vi "Alpha Ver 2.0.vi"() -> ()   [LabVIEW 2015]
uses:
  <instrlib>/Keithley 622x LV 2009/Utility/Typedefs/KE622x -- Instrument Type.ctl
  <instrlib>/Keithley 622x LV 2009/Keithley 622x.lvlib
panel:
  out "concatenated string":string
  out "write buffer":string="*RST\nSOUR:PDEL:HIGH 1e-3\nSOUR:PDEL:LOW 0\nSOUR:PDEL:WIDT 500e-6\nSOUR:PDEL:SDEL 100e-6\nSOUR:PDEL:COUN INF\nSOUR:PDEL:RANG BEST\nSOUR:PDEL:INT 5\nSOUR:PDEL:LME 2\nTRAC:POIN 200\nSOUR:PDEL:ARM\nINIT:IMM"
  out "LM_com":string
  out "I_com":string
  out "R_com":string
  out "C_com":string
  out "SD_com":string
  out "W_com":string
  out "LL_com":string
  out "HL_com":string
  in  "INF Button":bool
  in  "prefix 2":u16(ring)
  in  "prefix":u16(ring)
  in  "Low Measure":u16(ring)=1 items=["1", "2"]
  in  "Interval":dbl=5.0 min=5.0 max=999999.0 step=1.0
  in  "Ranging":string(combo)="BEST"
  in  "Count":dbl=1.0 min=1.0 max=65536.0 step=1.0
  in  "Source Delay":dbl
  in  "Width":dbl
  in  "Low Level":dbl min=-0.105 max=0.105
  in  "High Level":dbl
  out "2182A \nconnected ?":string
  in  "STOP":bool
  out "Measurement\nUnits":string
  out "2182A Voltage \nRange":string
  out "error out":errorcluster
  # "Pulse Measurement System"
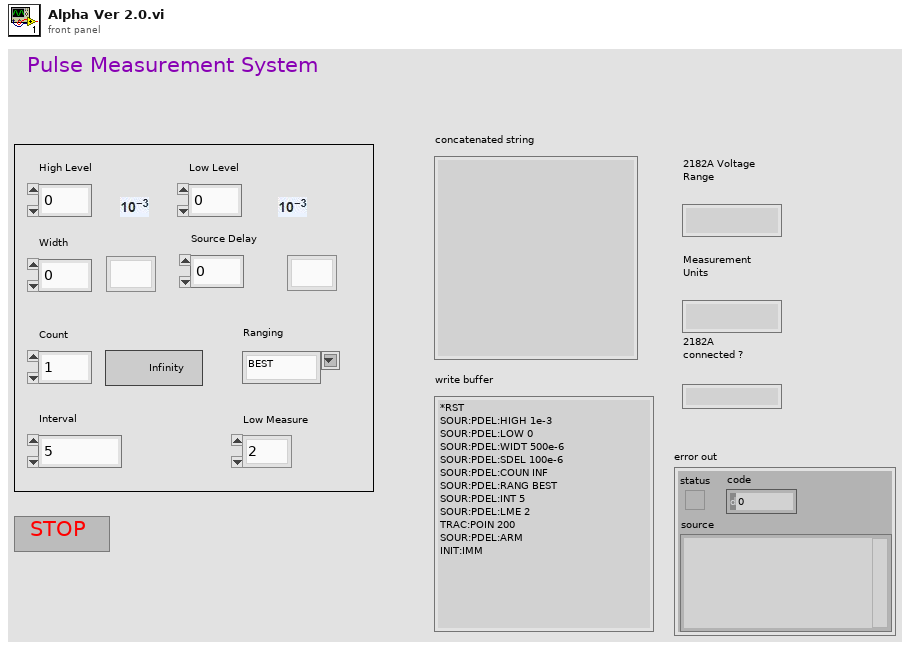
[diagram p1: front panel]
types:
  T1 = typedef "Keithley 622x.lvlib/KE622x -- Instrument Type.ctl" = enum16{"KE6220", "KE6221"}
  T2 = cluster{"VISA resource name out":refnum<visa-resource-name>, "error out":errorcluster}
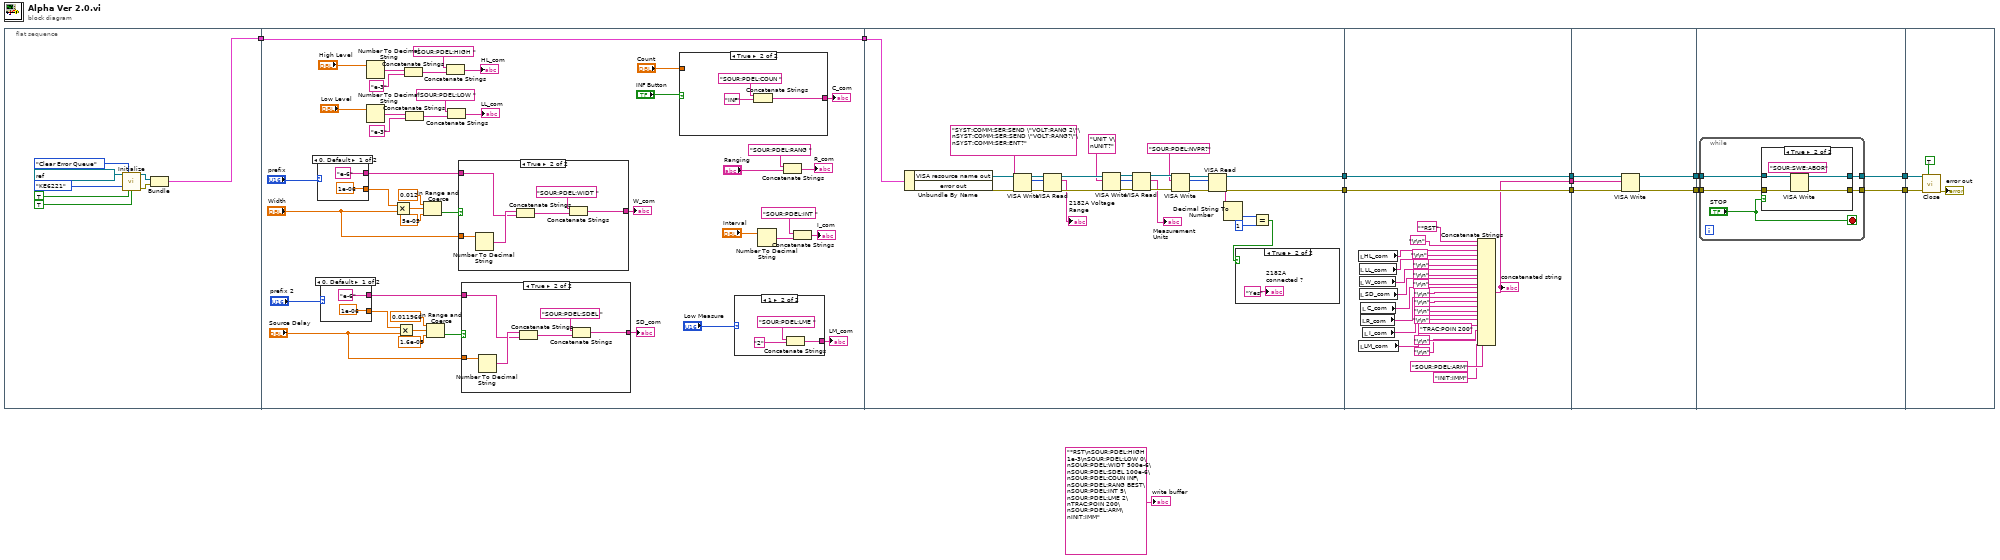
[diagram p0: block diagram]
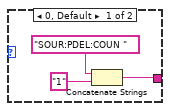
[diagram p2: hidden frame]
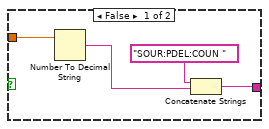
[diagram p3: hidden frame]
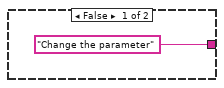
[diagram p4: hidden frame]
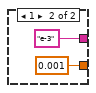
[diagram p5: hidden frame]
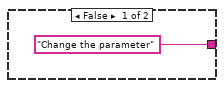
[diagram p6: hidden frame]
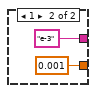
[diagram p7: hidden frame]
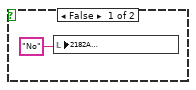
[diagram p8: hidden frame]
diagram:
  n1 = flat-sequence {
    tunnel: [w13] -> w8
    tunnel: w8 -> [w21]
    tunnel: [w21] -> w7
    tunnel: [w103] -> w6
    tunnel: [w102] -> w4
    tunnel: w7 -> [w101]
    tunnel: w6 -> [w153]
    tunnel: [w153] -> w5
    tunnel: w4 -> [w152]
    tunnel: [w152] -> w3
    tunnel: [w132] -> w1
    tunnel: w5 -> [w158]
    tunnel: [w157] -> w10
    tunnel: w3 -> [w156]
    tunnel: [w155] -> w9
    tunnel: w1 -> [w154]
    tunnel: w10 -> [w162]
    tunnel: w9 -> [w161]
    tunnel: [w160] -> w12
    tunnel: [w159] -> w11
    tunnel: w12 -> [w176]
    tunnel: w11 -> [w175]
    frame #0 {
      n2 = call <instrlib>:"Initialize.vi"("VISA resource name"=refnum<visa-resource-name> "Keithley_6221_2182A", "Error Queue Option"=enum16{"Clear Error Queue", "Error Query"}."Clear Error Queue", "Instrument Type"=KE622x_--_Instrument_Type."KE6221", "ID Query? (T)"=TRUE, "Reset? (T)"=TRUE) -> ("VISA resource name out"=w15:refnum<visa-resource-name>, "error out"=w14:errorcluster)  [unwired: 9 in]
      n3 = Bundle("VISA resource name out"=w15, "error out"=w14) -> (w13:T2)  [unwired: 1 in]
    }
    frame #1 {
      n4 = case shown="0, Default" "prefix" {
        tunnel: [1e-06 0.001] -> w44
        tunnel: ["e-6" ("string") "e-3" ("string")] -> w49
        frame 0, Default {
        }
        frame 1 {
        }
      }
      n5 = case shown="0, Default" "prefix 2" {
        tunnel: [1e-06 0.001] -> w39
        tunnel: ["e-6" ("string") "e-3" ("string")] -> w34
        frame 0, Default {
        }
        frame 1 {
        }
      }
      n6 = Number To Decimal String(number="High Level") -> (decimal integer string=w60:string)  [unwired: 1 in]
      n7 = Number To Decimal String(number="Low Level") -> (decimal integer string=w55:string)  [unwired: 1 in]
      n8 = Multiply(x=w44, y="Width") -> (x*y=w45:dbl)
      n9 = Multiply(x=w39, y="Source Delay") -> (x*y=w38:dbl)
      n10 = Concatenate Strings(w60, "e-3" ("string")) -> (w63:string)
      n11 = Concatenate Strings(w55, "e-3" ("string")) -> (w57:string)
      n12 = In Range and Coerce(upper limit=0.012, x=w45, lower limit=5e-05) -> (In Range?=w48:bool)  [unwired: 1 out]
      n13 = In Range and Coerce(upper limit=0.011966, x=w38, lower limit=1.6e-05) -> (In Range?=w35:bool)  [unwired: 1 out]
      n14 = Concatenate Strings("SOUR:PDEL:HIGH " ("string"), w63) -> (→"HL_com":string)
      n15 = Concatenate Strings("SOUR:PDEL:LOW " ("string"), w57) -> (→"LL_com":string)
      n16 = case shown="True" w48 {
        tunnel: w49 -> [_ w92]
        tunnel: "Width" -> [_ w94]
        tunnel: ["Change the parameter" w89] -> w51
        frame False {
        }
        frame True {
          n17 = Number To Decimal String(number=w94) -> (decimal integer string=w93:string)  [unwired: 1 in]
          n18 = Concatenate Strings(w93, w92) -> (w90:string)
          n19 = Concatenate Strings("SOUR:PDEL:WIDT " ("string"), w90) -> (w89:string)
        }
      }
      "W_com" <- w51
      n20 = case shown="True" w35 {
        tunnel: w34 -> [_ w81]
        tunnel: "Source Delay" -> [_ w83]
        tunnel: ["Change the parameter" w78] -> w42
        frame False {
        }
        frame True {
          n21 = Number To Decimal String(number=w83) -> (decimal integer string=w82:string)  [unwired: 1 in]
          n22 = Concatenate Strings(w82, w81) -> (w79:string)
          n23 = Concatenate Strings("SOUR:PDEL:SDEL " ("string"), w79) -> (w78:string)
        }
      }
      "SD_com" <- w42
      n24 = case shown="True" "INF Button" {
        tunnel: "Count" -> [w73 _]
        tunnel: [w71 w74] -> w33
        frame False {
          n25 = Number To Decimal String(number=w73) -> (decimal integer string=w70:string)  [unwired: 1 in]
          n26 = Concatenate Strings("SOUR:PDEL:COUN " ("string"), w70) -> (w71:string)
        }
        frame True {
          n27 = Concatenate Strings("SOUR:PDEL:COUN " ("string"), "INF") -> (w74:string)
        }
      }
      "C_com" <- w33
      n28 = case shown="1" "Low Measure" {
        tunnel: [w65 w67] -> w23
        frame 0, Default {
          n29 = Concatenate Strings("SOUR:PDEL:COUN " ("string"), "1" ("string")) -> (w65:string)
        }
        frame 1 {
          n30 = Concatenate Strings("SOUR:PDEL:LME " ("string"), "2") -> (w67:string)
        }
      }
      "LM_com" <- w23
      n31 = Number To Decimal String(number="Interval") -> (decimal integer string=w27:string)  [unwired: 1 in]
      n32 = Concatenate Strings("SOUR:PDEL:RANG " ("string"), "Ranging") -> (→"R_com":string)
      n33 = Concatenate Strings("SOUR:PDEL:INT " ("string"), w27) -> (→"I_com":string)
    }
    frame #2 {
      n34 = Unbundle By Name(w101) -> ("VISA resource name out"=w100:refnum<visa-resource-name>, "error out"=w99:errorcluster)
      n35 = VISA Write(VISA resource name=w100, write buffer="SYST:COMM:SER:SEND \"VOLT:RANG 2\"\nSYST:COMM:SER:SEND \"VOLT:RANG?\"\nSYST:COMM:SER:ENT?", error in (no error)=w99) -> (VISA resource name out=w123:refnum<visa-resource-name>, return count=w124:u32, error out=w122:errorcluster)
      n36 = VISA Read(VISA resource name=w123, byte count=w124, error in (no error)=w122) -> (VISA resource name out=w119:refnum<visa-resource-name>, read buffer=→"2182A Voltage \nRange":string, error out=w121:errorcluster)  [unwired: 1 out]
      n37 = VISA Write(VISA resource name=w119, write buffer="UNIT V\nUNIT?", error in (no error)=w121) -> (VISA resource name out=w115:refnum<visa-resource-name>, return count=w116:u32, error out=w117:errorcluster)
      n38 = VISA Read(VISA resource name=w115, byte count=w116, error in (no error)=w117) -> (VISA resource name out=w112:refnum<visa-resource-name>, read buffer=→"Measurement\nUnits":string, error out=w114:errorcluster)  [unwired: 1 out]
      n39 = VISA Write(VISA resource name=w112, write buffer="SOUR:PDEL:NVPR?", error in (no error)=w114) -> (VISA resource name out=w108:refnum<visa-resource-name>, return count=w109:u32, error out=w110:errorcluster)
      n40 = VISA Read(VISA resource name=w108, byte count=w109, error in (no error)=w110) -> (VISA resource name out=w103:refnum<visa-resource-name>, read buffer=w106:string, error out=w102:errorcluster)  [unwired: 1 out]
      n41 = Decimal String To Number(string=w106) -> (number=w105:i32)  [unwired: 2 in, 1 out]
      n42 = Equal?(x=w105, y=1) -> (x = y?=w107:bool)
      n43 = case shown="True" w107 {
        frame False {
          n44 = local write "2182A \nconnected ?"("No" ("2182A \nconnected ?")) -> ()
        }
        frame True {
          "2182A \nconnected ?" <- "Yes" ("2182A \nconnected ?")
        }
      }
    }
    frame #3 {
      n45 = local read "HL_com"() -> (w149:string)
      n46 = local read "LM_com"() -> (w135:string)
      n47 = local read "LL_com"() -> (w147:string)
      n48 = local read "W_com"() -> (w145:string)
      n49 = local read "SD_com"() -> (w143:string)
      n50 = local read "R_com"() -> (w140:string)
      n51 = local read "C_com"() -> (w141:string)
      n52 = local read "I_com"() -> (w137:string)
      n53 = Concatenate Strings("*RST" ("string"), "\r\n", w149, "\r\n", w147, "\r\n", w145, "\r\n", w143, "\r\n", w141, "\r\n", w140, "\r\n", w137, "\r\n", w135, "\r\n", "TRAC:POIN 200" ("string"), "\r\n", "SOUR:PDEL:ARM" ("string"), "\r\n", "INIT:IMM" ("string")) -> (w132:string)
      "concatenated string" <- w132
    }
    frame #4 {
      n54 = VISA Write(VISA resource name=w158, write buffer=w154, error in (no error)=w156) -> (VISA resource name out=w157:refnum<visa-resource-name>, error out=w155:errorcluster)  [unwired: 1 out]
    }
    frame #5 {
      n55 = while {
        tunnel: w162 -> [w167]
        tunnel: w161 -> [w166]
        tunnel: [w164] -> w160
        tunnel: [w163] -> w159
        stop <- "STOP" stop-if-true
        n56 = case shown="True" "STOP" {
          tunnel: w167 -> [w168 w173]
          tunnel: w166 -> [w169 w172]
          tunnel: [w168 w171] -> w164
          tunnel: [w169 w170] -> w163
          frame False {
          }
          frame True {
            n57 = VISA Write(VISA resource name=w173, write buffer="SOUR:SWE:ABOR", error in (no error)=w172) -> (VISA resource name out=w171:refnum<visa-resource-name>, error out=w170:errorcluster)  [unwired: 1 out]
          }
        }
      }
    }
    frame #6 {
      n58 = call <instrlib>:"Close.vi"("VISA resource name"=w176, "Query For SCPI Errors? (T)"=TRUE, "error in (no error)"=w175) -> ("error out"=→"error out":errorcluster)  [unwired: 12 in]
    }
  }
  "write buffer" <- "*RST\nSOUR:PDEL:HIGH 1e-3\nSOUR:PDEL:LOW 0\nSOUR:PDEL:WIDT 500e-6\nSOUR:PDEL:SDEL 100e-6\nSOUR:PDEL:COUN INF\nSOUR:PDEL:RANG BEST\nSOUR:PDEL:INT 5\nSOUR:PDEL:LME 2\nTRAC:POIN 200\nSOUR:PDEL:ARM\nINIT:IMM" ("write buffer")
